vi "Append User Formatted HTML to Report.vi"(4 "error in (no error)":errorcluster, 6 "HTML text":string, 7 "report in":T1) -> (0 "error out":errorcluster, 3 "report out":T1)   [LabVIEW 2015]
doc: "Inserts text that is not LabVIEW preformatted in the HTML report. You cannot use this VI with standard reports."
uses:
  <vilib>/Utility/NIReport.llb/Generate Report Object Reference.ctl
  <vilib>/Utility/NIReport.llb/NI_report.lvclass
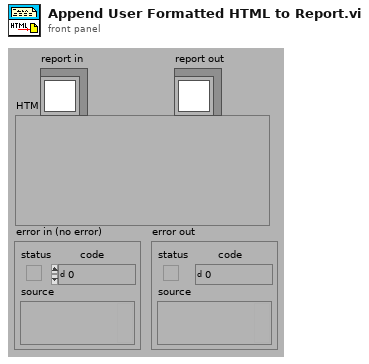
[diagram p1: front panel]
types:
  T1 = typedef "Generate Report Object Reference.ctl" = refnum<class "NI_report.lvclass">
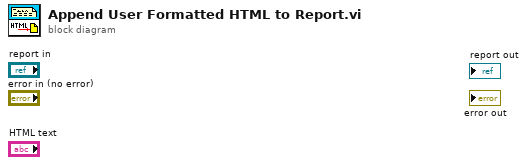
[diagram p0: block diagram]
diagram:
